vi "ExampleMessageFGV.vi"() -> ()   [LabVIEW 2019, in "MicronTemplateAPIs.lvlib" / "MicronTemplateAPIs.lvclass"]
uses:
  MicronTemplateAPIs.lvclass
  9ceadd3c-745e-4cc0-becc-c9896ef65399.vi
panel:
  in  "Stop?":bool
  out "error out":errorcluster
  out "Response":string
  in  "Command":string="Hello Micron!"
  in  "Payload":string="An Open Source Microservice Architecture on top of gRPC from https://github.com/KarthikAbiram/Micron"
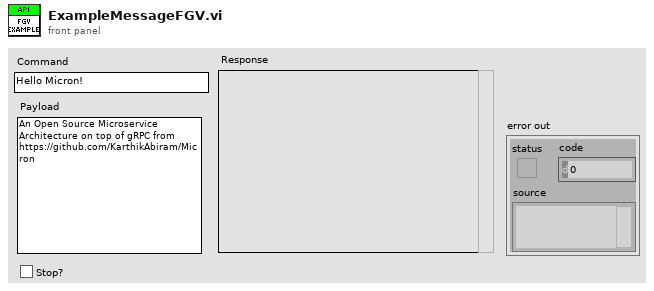
[diagram p1: front panel]
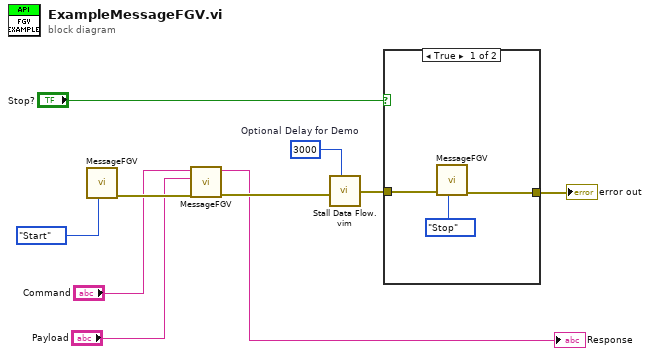
[diagram p0: block diagram]
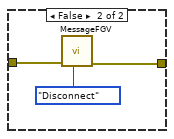
[diagram p2: hidden frame]
diagram:
  w10 = u32 3000  # Optional Delay for Demo
  n1 = call "MessageFGV.vi"("Operation"=enum16{"Start", "Message", "Stop", "Disconnect"}."Start") -> ("error out"=w9:errorcluster)  [unwired: 9 in, 1 out]
  n2 = call "MessageFGV.vi"("error in (no error)"=w9, "Payload"="Payload", "Command"="Command") -> ("error out"=w7:errorcluster, "Response"=→"Response":string)  [unwired: 7 in]
  n3 = call "Stall Data Flow.vim"("value in"=w7, "milliseconds to wait"=w10) -> ("value out"=w6:errorcluster)  [unwired: 1 out]
  n4 = case shown="True" "Stop?" {
    tunnel: w6 -> [w13 w16]
    tunnel: [w12 w15] -> w2
    frame True {
      n5 = call "MessageFGV.vi"("Operation"=enum16{"Start", "Message", "Stop", "Disconnect"}."Stop", "error in (no error)"=w13) -> ("error out"=w12:errorcluster)  [unwired: 8 in, 1 out]
    }
    frame False {
      n6 = call "MessageFGV.vi"("Operation"=enum16{"Start", "Message", "Stop", "Disconnect"}."Disconnect", "error in (no error)"=w16) -> ("error out"=w15:errorcluster)  [unwired: 8 in, 1 out]
    }
  }
  "error out" <- w2
